vi "QTrkGetResultCount.vi"(4 "error in (no error)":errorcluster, 7 "QTrk Instance":T1) -> (0 "error out":errorcluster, 2 "result count":i32, 3 "QTrk Instance":T1)   [LabVIEW 2011]
uses:
  QTrkInstance.ctl
  QTrkDLL.vi
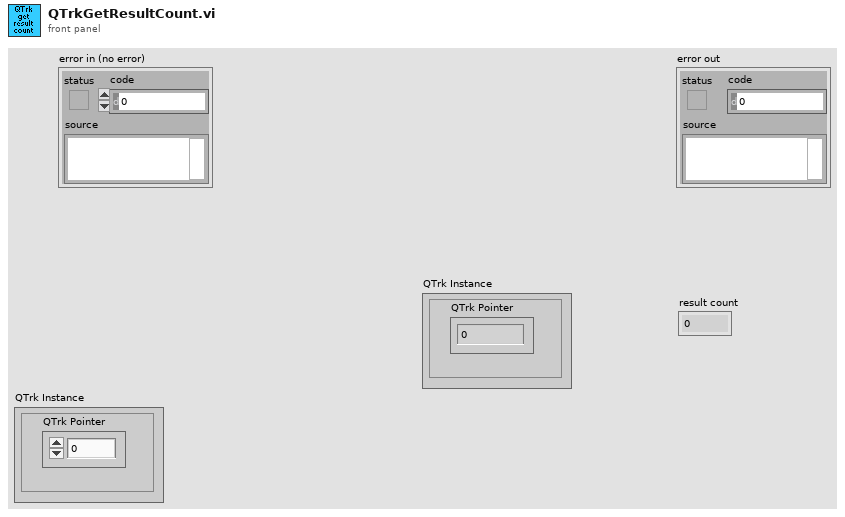
[diagram p1: front panel]
types:
  T1 = typedef "QTrkInstance.ctl" = cluster{"QTrk Pointer":u64}
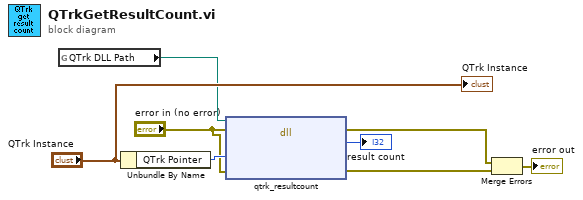
[diagram p0: block diagram]
diagram:
  n1 = global read "QTrkDLL.vi" "QTrk DLL Path"() -> (w6:path)
  n2 = Unbundle By Name("QTrk Instance") -> ("QTrk Pointer"=w7:u64)
  n3 = dll-call lib="D:/jcnossen1/cudaqi-tracker/bin/jtrk-labview.dll" fn="qtrk_resultcount"(path in=w6, error in="error in (no error)", "tracker"=w7, "error"="error in (no error)") -> (error out=w2:errorcluster, "result count"=→"result count":i32, "error"=w3:errorcluster)  [unwired: 2 in, 1 out]
  n4 = Merge Errors(w2, w3) -> (→"error out":errorcluster)
  "QTrk Instance" <- "QTrk Instance"
